vi "Parameter1.vi"(5 "继承模式":string, 7 "模式":enum16{"select", "insert", "update", "delete"}(ring), 10 "dataIn":T1={"productsName"="", "parameterName"="", "unit"="", "result"="", "vaule"=nan, "limitH"=nan, "limitL"=nan}) -> (2 "dataOutAll":T2(array[cluster]))   [LabVIEW 2012]
uses:
  <vilib>/addons/database/Auxilliary.llb/DB Tools Parameter Info.ctl
  <vilib>/addons/database/Auxilliary.llb/DB Tools DataTypes.ctl
  <vilib>/addons/database/Auxilliary.llb/DB Tools Parameter Dir.ctl
  <vilib>/addons/database/_DB Variant To Data/Database Variant To Data.xnode
  <vilib>/addons/database/NI_Database_API.lvlib
  <vilib>/Utility/VariantDataType/VariantType.lvlib
panel:
  out "SQL query":string
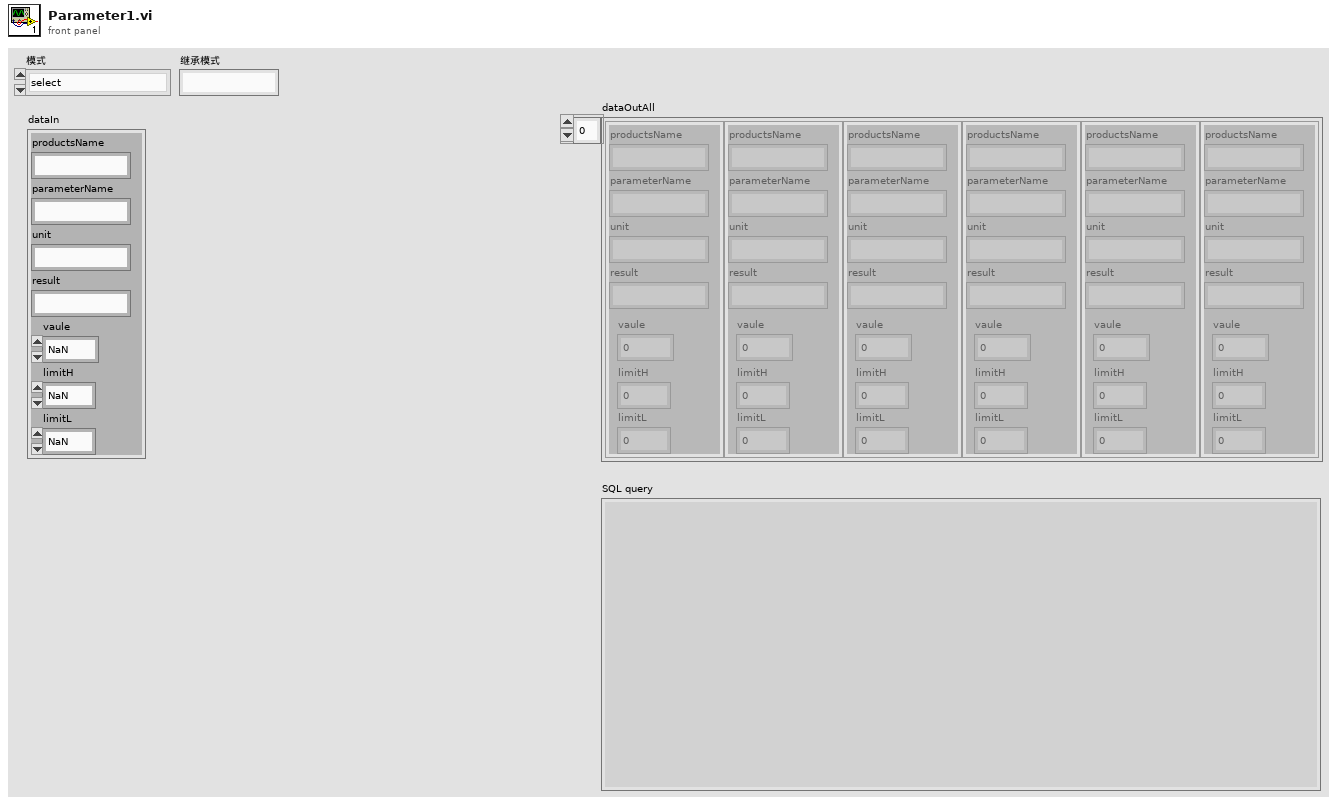
[diagram p1: front panel]
types:
  T1 = cluster{"productsName":string, "parameterName":string, "unit":string, "result":string, "vaule":dbl, "limitH":dbl, "limitL":dbl}
  T2 = cluster{"productsName":string, "parameterName":string, "unit":string, "result":string, "vaule":dbl, "limitH":dbl, "limitL":dbl}[]
  T3 = cluster{"productsName":string, "parameterName":string, "unit":string, "result":string, "vaule":string, "limitH":string, "limitL":string}[]
  T4 = typedef "NI_Database_API.lvlib/DB Tools Parameter Info.ctl" = cluster{"parameter name":string, "type":T5, "direction":T6, "value":variant}
  T5 = typedef "NI_Database_API.lvlib/DB Tools DataTypes.ctl" = enum16{"String", "Long (I32)", "Single (SGL)", "Double (DBL)", "Date/Time", "Binary"}
  T6 = typedef "NI_Database_API.lvlib/DB Tools Parameter Dir.ctl" = enum32{"Input", "Output", "Input/Output", "Return Value"}
  T7 = typedef "VariantType.lvlib/Type.ctl" = enum8{"Invalid Type", "Void", "I8", "I16", "I32", "I64", "U8", "U16", "U32", "U64", "Single Float", "Double Float", "Extended Float", "Single Complex", "Double Complex", "Extended Complex", "Enum U8", "Enum U16", "Enum U32", "Enum U64", "Single Float With Unit", "Double Float With Unit", "Extended Float With Unit", "Single Complex with Unit", "Double Complex with Unit", "Extended Complex with Unit", "Boolean", "String", "Path", "Picture", "Tag", "Array", "Cluster", "Variant", "LV Variant", "Waveform", "Timestamp", "Digital Waveform", "Digital Data", "ExpressData", "Refnum", "External Data", "VI", "Poly VI", "LabVIEW Class Instance", "Fixed Point"}
  T8 = cluster{"productsName":string, "parameterName":string, "unit":string, "result":string, dbl, dbl, dbl}
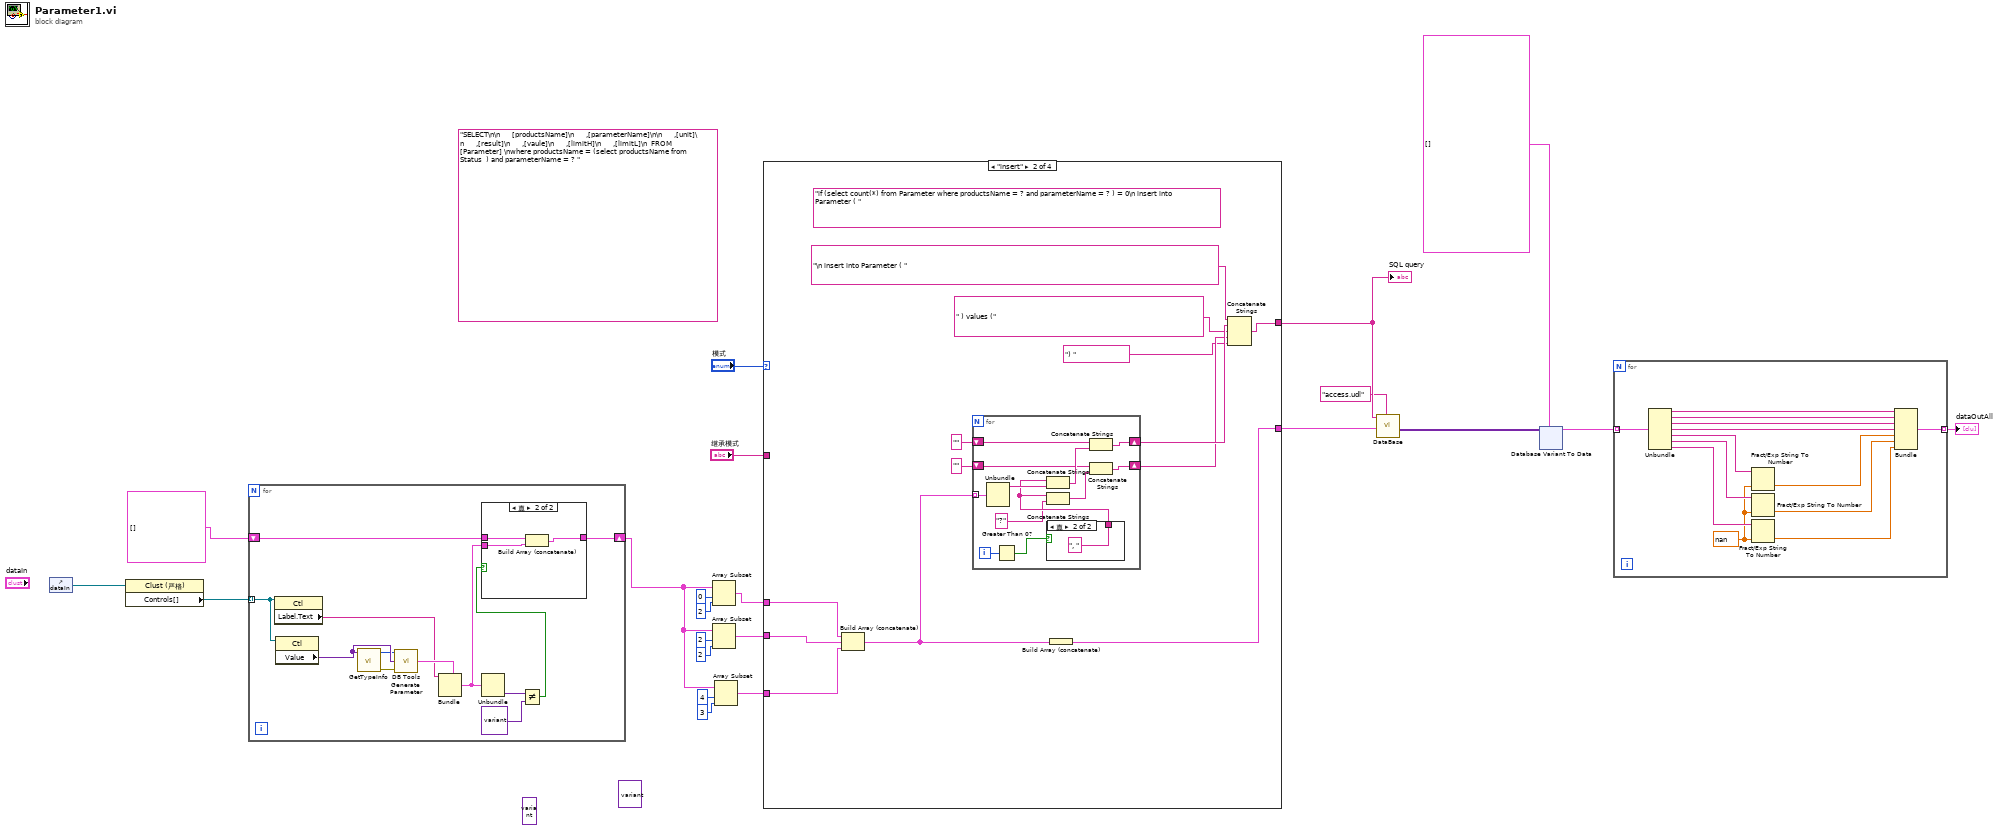
[diagram p0: block diagram]
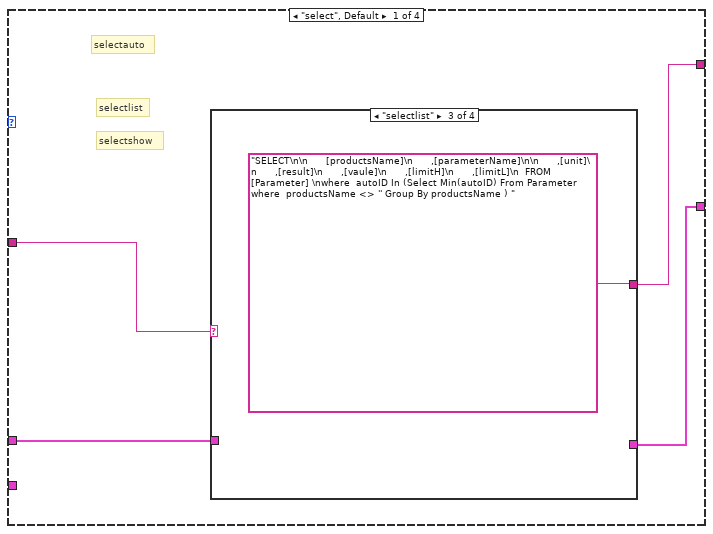
[diagram p3: hidden frame]
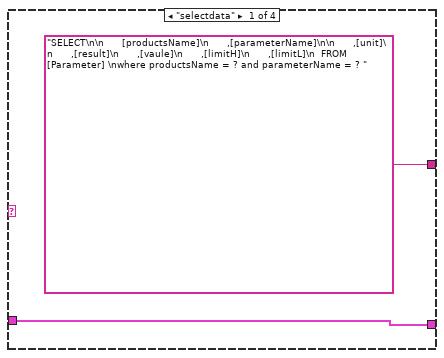
[diagram p4: hidden frame]
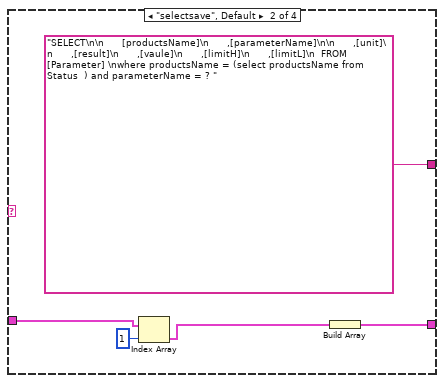
[diagram p5: hidden frame]
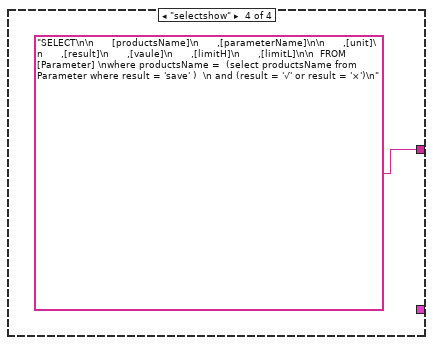
[diagram p6: hidden frame]
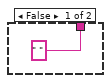
[diagram p7: hidden frame]
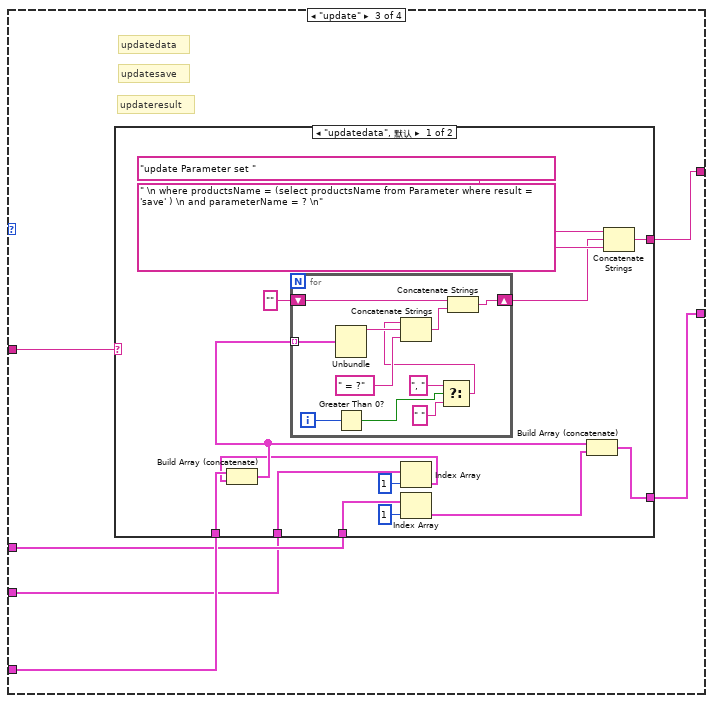
[diagram p8: hidden frame]
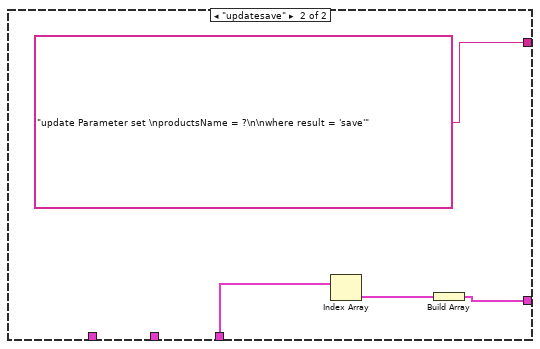
[diagram p9: hidden frame]
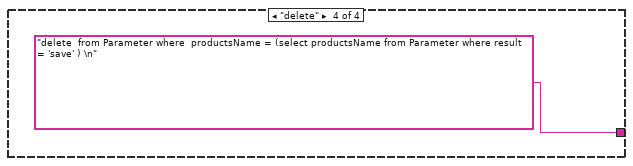
[diagram p10: hidden frame]
diagram:
  (unwired) "SELECT\n\n      [productsName]\n      ,[parameterName]\n\n      ,[unit]\n      ,[result]\n      ,[vaule]\n      ,[limitH]\n      ,[limitL]\n  FROM [Parameter] \nwhere productsName = (select productsName from Status  ) and parameterName = ? " ("SQL query")
  (unwired) variant(string "") ("变体")
  (unwired) variant(string "all") ("value")
  n1 = control-ref of="dataIn"() -> (w5:refnum<vi>)
  n2 = property on="属性节点" class="Clust (严格)"(reference=w5) -> ("Controls[]"=w6:refnum<vi>[])  [unwired: 1 in, 2 out]
  n3 = for {
    tunnel: w6 -> [w34] mode=indexing
    shift-right: [w27] -> w10
    shift-left: T4[] [] ("添加的数组") -> [w28]
    n4 = property on="属性节点" class="Ctl"(reference=w34) -> ("Label.Text"=w29:string)  [unwired: 1 in, 2 out]
    n5 = property on="属性节点" class="Ctl"(reference=w34) -> ("Value"=w33:variant)  [unwired: 1 in, 2 out]
    n6 = call <vilib>:"GetTypeInfo.vi"("Variant"=w33) -> ("error out"=w31:errorcluster, "Type Enum"=w32:T7)  [unwired: 6 in, 3 out]
    n7 = call <vilib>:"DB Tools Generate Parameter.vi"("Type Enum"=w32, "Variant data"=w33, "error in (no error)"=w31) -> ("parameter information"=w30:T4)  [unwired: 11 in, 1 out]
    n8 = Bundle(cluster=w30, "parameter name"=w29) -> (w23:T4)  [unwired: 3 in]
    n9 = Unbundle(w23) -> ("value"=w26:variant)  [unwired: 3 out]
    n10 = Not Equal?(x=w26, y=variant(dbl nan) ("value")) -> (x != y?=w24:bool)
    n11 = case shown="真" w24 {
      tunnel: w28 -> [w35 w38]
      tunnel: [w35 w37] -> w27
      tunnel: w23 -> [_ w36]
      frame False {
      }
      frame True {
        n12 = Build Array (concatenate)(w38, w36) -> (w37:T4[])
      }
    }
  }
  n13 = Array Subset(array=w10, index=0 ("索引"), length=2 ("长度")) -> (w14:T4[])
  n14 = Array Subset(array=w10, index=2 ("索引"), length=2 ("长度")) -> (w9:T4[])
  n15 = Array Subset(array=w10, index=4 ("索引"), length=3 ("长度")) -> (w15:T4[])
  n16 = case shown="\"insert\"" "模式" {
    tunnel: [w41 w52 w82 _] -> w21
    tunnel: [w42 w57 w84 "delete  from Parameter where  productsName = (select productsName from Parameter where result = 'save' ) \n" ("SQL query")] -> w13
    tunnel: w14 -> [w39 w53 w81 _]
    tunnel: w15 -> [_ w55 w83 _]
    tunnel: w9 -> [_ w56 w79 _]
    tunnel: "继承模式" -> [w40 _ w80 _]
    frame "select", Default {
      # "selectshow"
      # "selectauto"
      # "selectlist"
      n17 = case shown="\"selectlist\"" w40 {
        tunnel: ["SELECT\n\n      [productsName]\n      ,[parameterName]\n\n      ,[unit]\n      ,[result]\n      ,[vaule]\n      ,[limitH]\n      ,[limitL]\n  FROM [Parameter] \nwhere productsName = ? and parameterName = ? " ("SQL query") "SELECT\n\n      [productsName]\n      ,[parameterName]\n\n      ,[unit]\n      ,[result]\n      ,[vaule]\n      ,[limitH]\n      ,[limitL]\n  FROM [Parameter] \nwhere productsName = (select productsName from Status  ) and parameterName = ? " ("SQL query") "SELECT\n\n      [productsName]\n      ,[parameterName]\n\n      ,[unit]\n      ,[result]\n      ,[vaule]\n      ,[limitH]\n      ,[limitL]\n  FROM [Parameter] \nwhere  autoID In (Select Min(autoID) From Parameter  where  productsName <> '' Group By productsName ) " ("SQL query") "SELECT\n\n      [productsName]\n      ,[parameterName]\n\n      ,[unit]\n      ,[result]\n      ,[vaule]\n      ,[limitH]\n      ,[limitL]\n\n  FROM [Parameter] \nwhere productsName =  (select productsName from Parameter where result = 'save' )  \n and (result = '√' or result = '×')\n" ("SQL query")] -> w42
        tunnel: [w43 w48 _ _] -> w41
        tunnel: w39 -> [w43 w46 _ _]
        frame "selectdata" {
        }
        frame "selectsave", Default {
          n18 = Index Array(array=w46, index=1 ("索引")) -> (element=w45:T4)
          n19 = Build Array(w45) -> (w48:T4[])
        }
        frame "selectlist" {
        }
        frame "selectshow" {
        }
      }
    }
    frame "insert" {
      (unwired) "if (select count(*) from Parameter where productsName = ? and parameterName = ? ) = 0\n insert into Parameter ( " ("SQL query")
      n20 = Build Array (concatenate)(w53, w56, w55) -> (w54:T4[])
      n21 = for {
        tunnel: w54 -> [w76] mode=indexing
        shift-right: [w73] -> w61
        shift-left: "" ("SQL query") -> [w74]
        shift-right: [w68] -> w59
        shift-left: "" ("SQL query") -> [w70]
        i -> [w71]
        n22 = Unbundle(w76) -> ("parameter name"=w75:string)  [unwired: 3 out]
        n23 = Greater Than 0?(x=w71) -> (x > 0?=w69:bool)
        n24 = case shown="真" w69 {
          tunnel: [" " ("字符串") ", " ("字符串")] -> w66
          frame False {
          }
          frame True {
          }
        }
        n25 = Concatenate Strings(w66, w75) -> (w72:string)
        n26 = Concatenate Strings(w66, "?" ("字符串")) -> (w67:string)
        n27 = Concatenate Strings(w74, w72) -> (w73:string)
        n28 = Concatenate Strings(w70, w67) -> (w68:string)
      }
      n29 = Build Array (concatenate)(w54) -> (w52:T4[])
      n30 = Concatenate Strings("\n insert into Parameter ( " ("SQL query"), w61, " ) values (" ("SQL query"), w59, ") " ("SQL query")) -> (w57:string)
    }
    frame "update" {
      # "updatedata"
      # "updatesave"
      # "updateresult"
      n31 = case shown="\"updatedata\", 默认" w80 {
        tunnel: [w97 "update Parameter set \nproductsName = ?\n\nwhere result = 'save'" ("SQL query")] -> w84
        tunnel: w83 -> [w87 _]
        tunnel: [w93 w111] -> w82
        tunnel: w81 -> [w91 w113]
        tunnel: w79 -> [w89 _]
        frame "updatedata", Default {
          n32 = Index Array(array=w89, index=1 ("索引")) -> (element=w85:T4)
          n33 = Build Array (concatenate)(w87, w85) -> (w88:T4[])
          n34 = for {
            tunnel: w88 -> [w109] mode=indexing
            shift-right: [w105] -> w95
            shift-left: "" ("SQL query") -> [w106]
            i -> [w103]
            n35 = Unbundle(w109) -> ("parameter name"=w108:string)  [unwired: 3 out]
            n36 = Greater Than 0?(x=w103) -> (x > 0?=w100:bool)
            n37 = Select(t=", " ("字符串"), s=w100, f=" " ("字符串")) -> (s? t:f=w99:string)
            n38 = Concatenate Strings(w99, w108, " = ?" ("SQL query")) -> (w104:string)
            n39 = Concatenate Strings(w106, w104) -> (w105:string)
          }
          n40 = Index Array(array=w91, index=1 ("索引")) -> (element=w86:T4)
          n41 = Build Array (concatenate)(w88, w86) -> (w93:T4[])
          n42 = Concatenate Strings("update Parameter set " ("SQL query"), w95, " \n where productsName = (select productsName from Parameter where result = 'save' ) \n and parameterName = ? \n" ("SQL query")) -> (w97:string)
        }
        frame "updatesave" {
          n43 = Index Array(array=w113) -> (element=w112:T4)  [unwired: 1 in]
          n44 = Build Array(w112) -> (w111:T4[])
        }
      }
    }
    frame "delete" {
    }
  }
  "SQL query" <- w13
  n45 = call "DataBase.vi"("udl名称"="access.udl", "parameters"=w21, "SQL query"=w13) -> ("recordset data"=w8:variant[][])  [unwired: 8 in]
  n46 = xnode ("Database Variant To Data")("database variant"=w8, "type"=T3 [] ("添加的数组")) -> ("data"=w7:T3)  [unwired: 1 in, 1 out]
  n47 = for {
    tunnel: w7 -> [w127] mode=indexing
    tunnel: [w115] -> w2 mode=indexing
    w123 = nan ("默认(0 DBL)")
    n48 = Unbundle(w127) -> ("productsName"=w122:string, "parameterName"=w121:string, "unit"=w120:string, "result"=w119:string, "vaule"=w126:string, "limitH"=w125:string, "limitL"=w124:string)
    n49 = Fract/Exp String To Number(string=w126, default (0 dbl)=w123) -> (number=w118:dbl)  [unwired: 2 in, 1 out]
    n50 = Fract/Exp String To Number(string=w125, default (0 dbl)=w123) -> (number=w117:dbl)  [unwired: 2 in, 1 out]
    n51 = Fract/Exp String To Number(string=w124, default (0 dbl)=w123) -> (number=w116:dbl)  [unwired: 2 in, 1 out]
    n52 = Bundle("productsName"=w122, "parameterName"=w121, "unit"=w120, "result"=w119, w118, w117, w116) -> (w115:T8)  [unwired: 1 in]
  }
  "dataOutAll" <- w2
